vi "Laser Power Ctrl Ext Setup.vi"(0 "Wavelength":u16, 7 "Previous Path":path, 11 "Settings":string[](array[string])) -> (4 "Settings Out":string[](array[string]), 8 "Ext Ctrl Path":path, 15 "Canceled?":bool)   [LabVIEW 2020]
uses:
  <vilib>/Utility/miscctls.llb/LVPointTypeDef.ctl
panel:
  in  "Select Source":bool
  in  "Calling VI Ref":refnum<vi>
  in  "Cancel":bool
  in  "Done":bool
  in  "Setting 10":string
  in  "Setting 09":string
  in  "Setting 08":string
  in  "Setting 07":string
  in  "Setting 06":string
  in  "Setting 05":string
  in  "Setting 04":string
  in  "Setting 03":string
  in  "Setting 02":string
  in  "Setting 01":string
  out "External Power Control VI":string
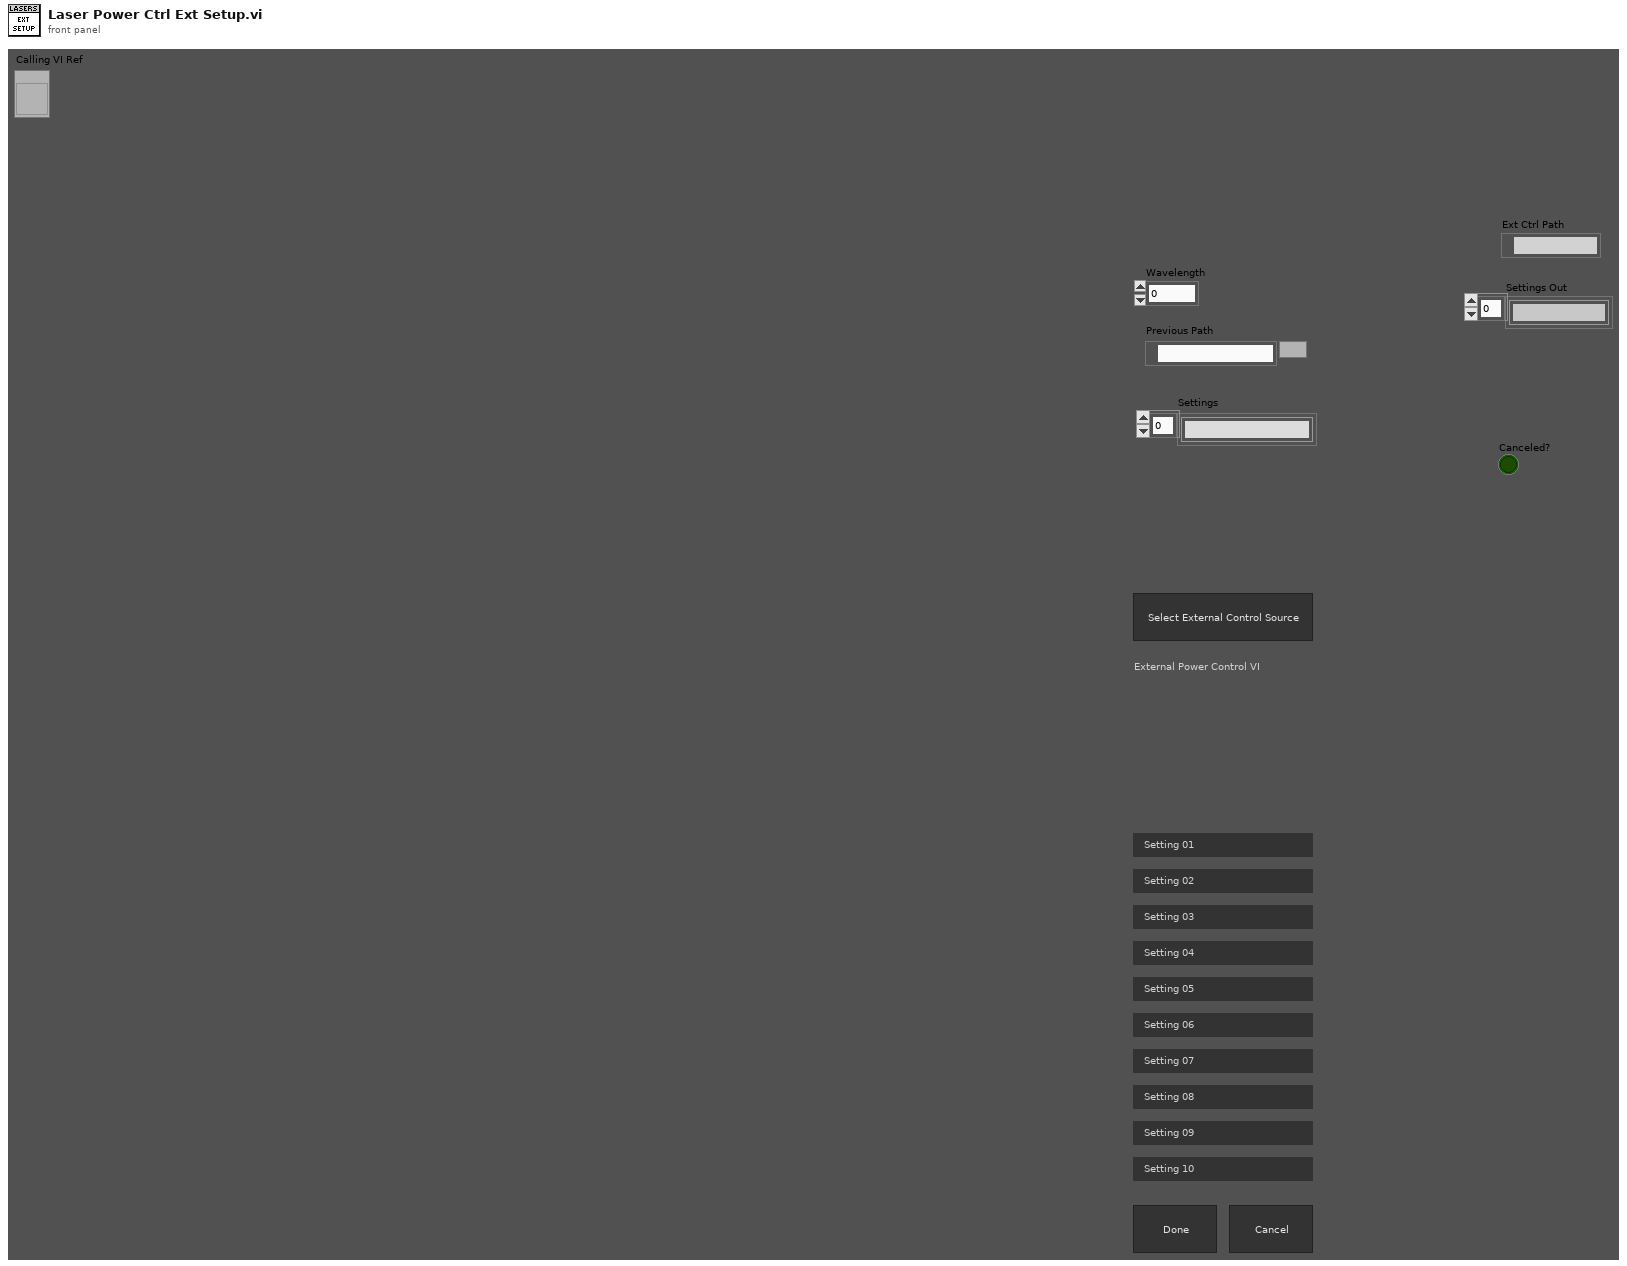
[diagram p1: front panel]
types:
  T1 = enum16{"Always On", "Always Off", "Off While Running"}
  T2 = typedef "LVPointTypeDef.ctl" = cluster{"Horizontal":i16, "Vertical":i16}
  T3 = typedef "LVRectTypeDef.ctl" = cluster{"Left":i16, "Top":i16, "Right":i16, "Bottom":i16}
  T4 = typedef "LVBoundsTypeDef.ctl" = cluster{"Width":u32, "Height":u32}
  T5 = enum8{"Enabled", "Disabled", "Disabled and Grayed Out"}
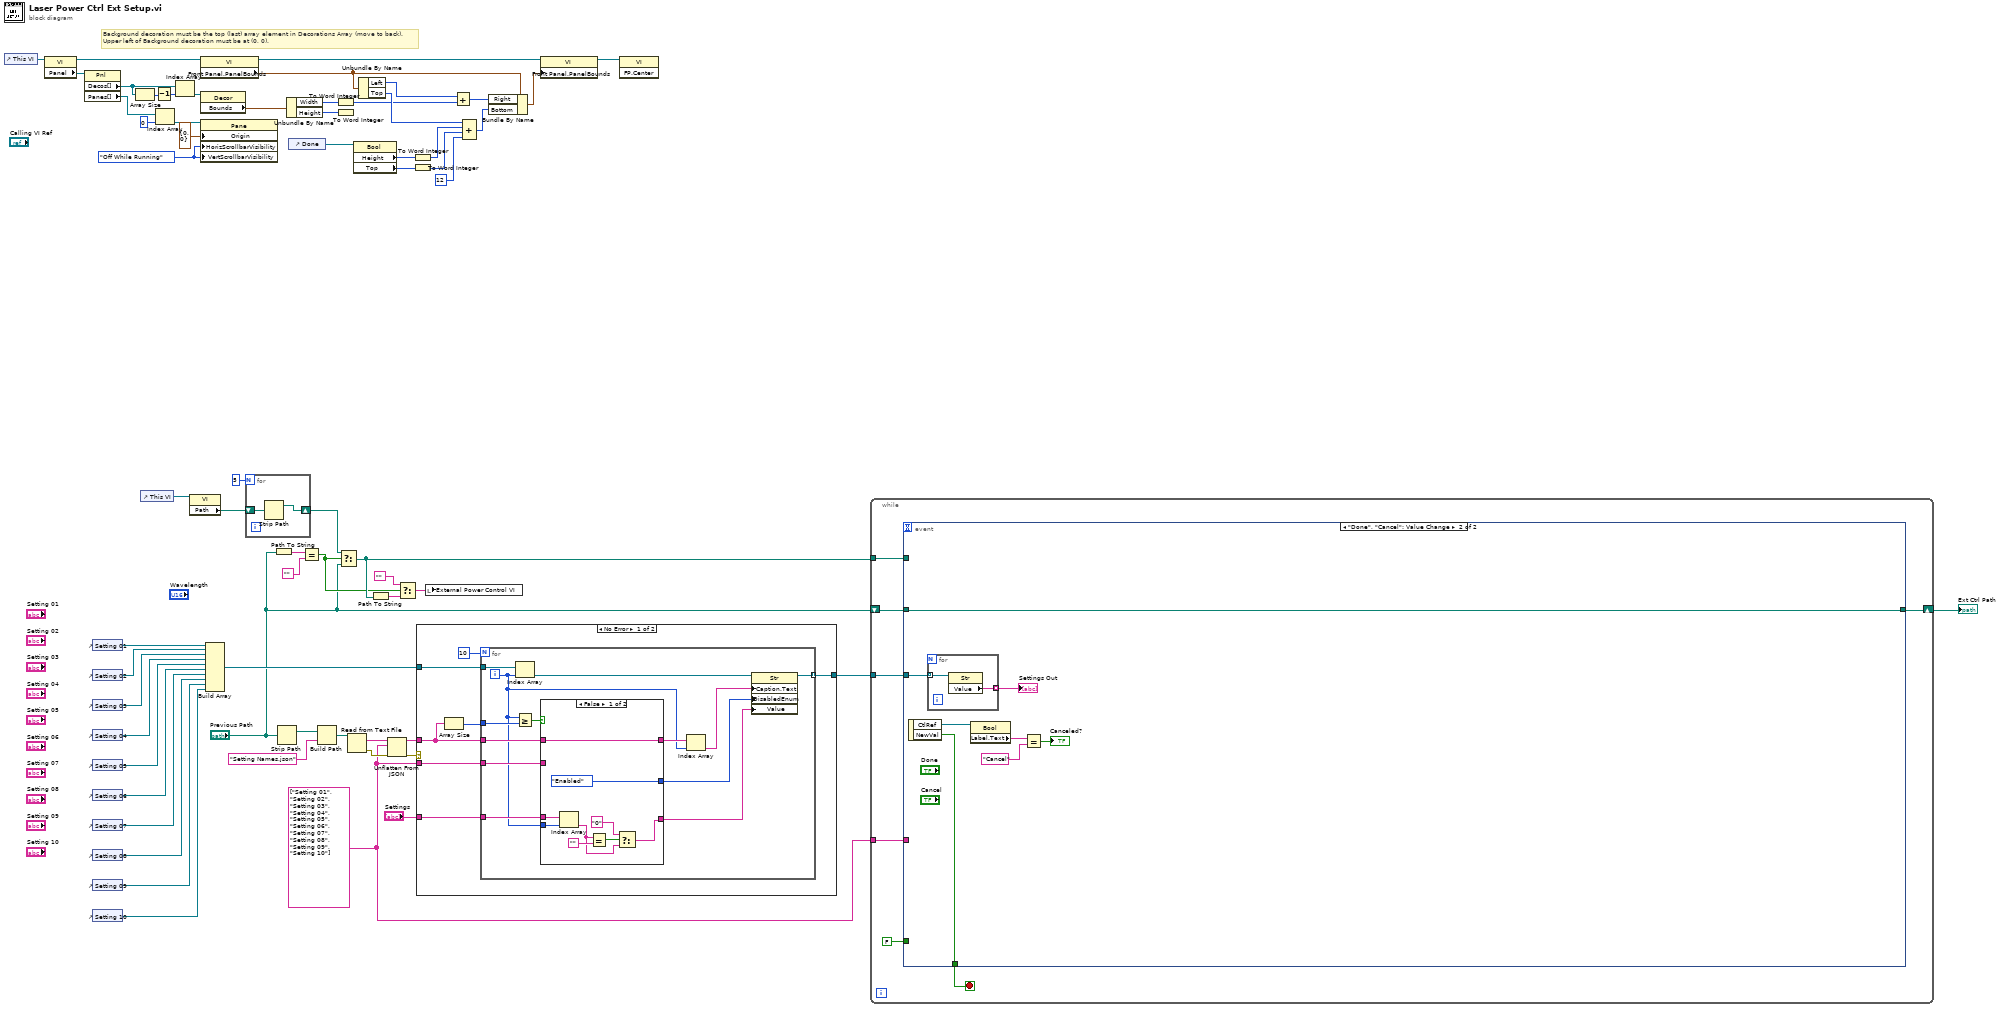
[diagram p0: block diagram]
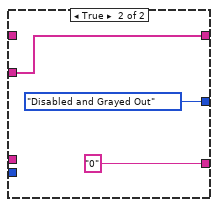
[diagram p2: hidden frame]
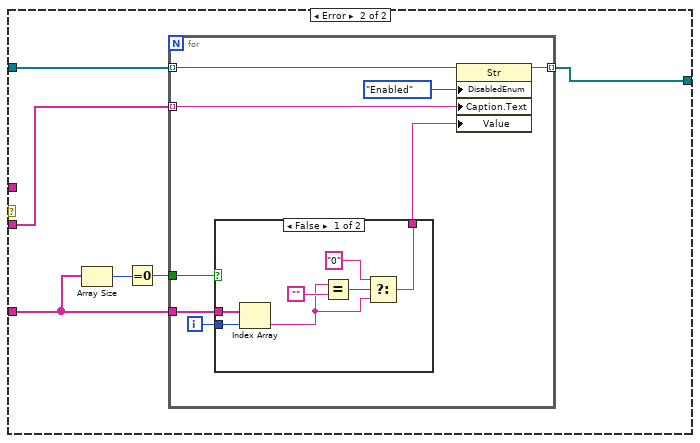
[diagram p3: hidden frame]
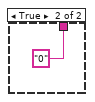
[diagram p4: hidden frame]
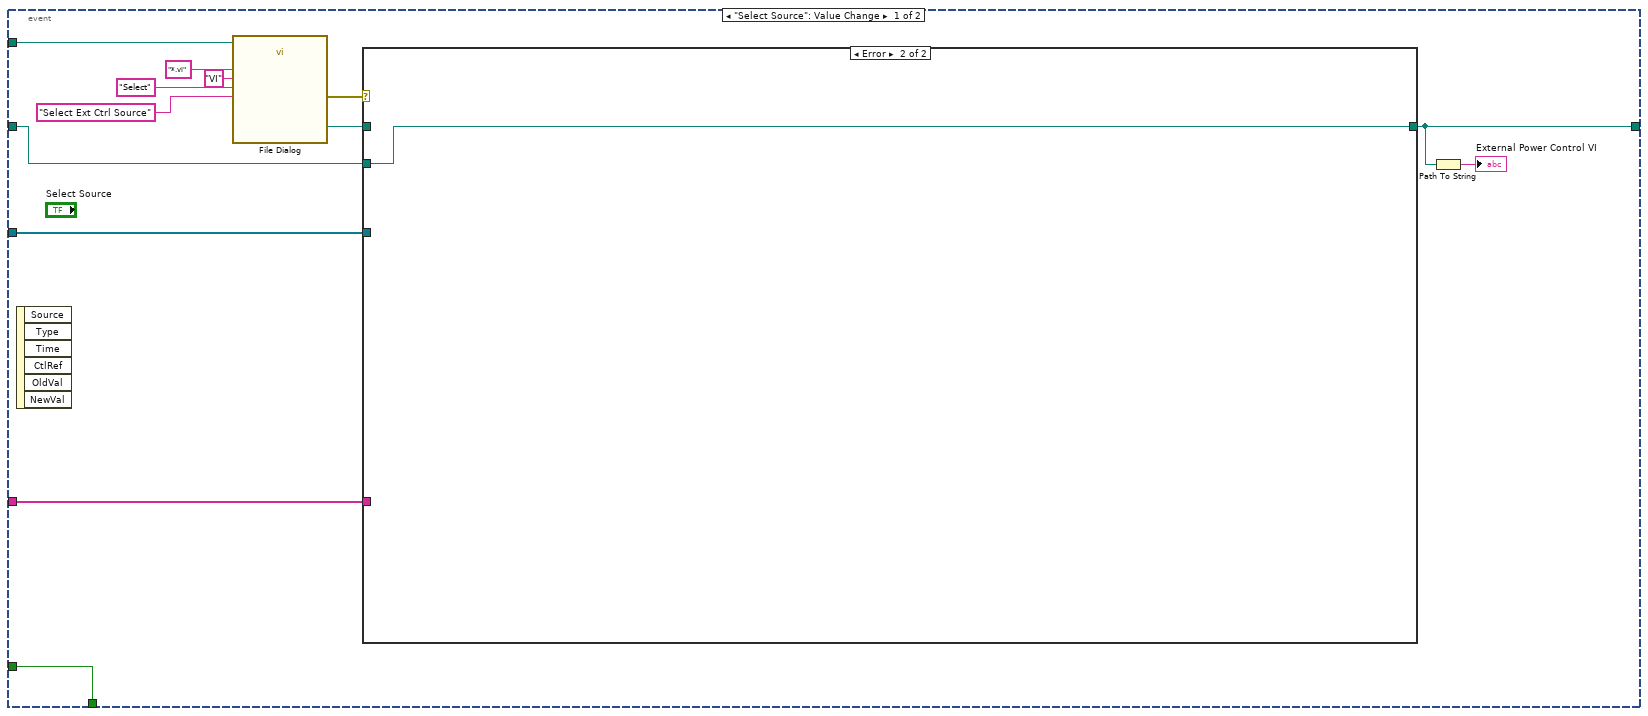
[diagram p5: hidden frame]
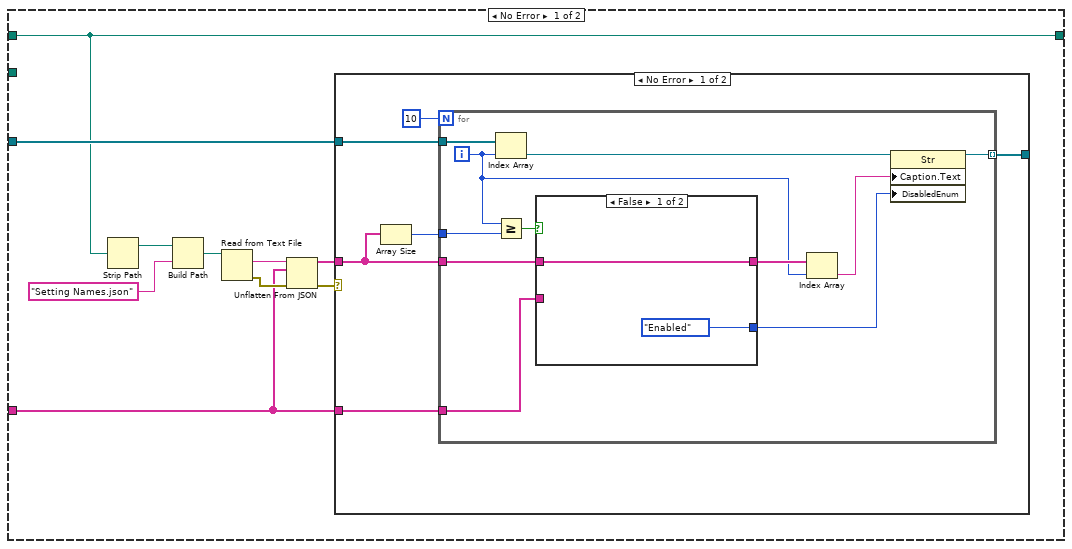
[diagram p6: hidden frame]
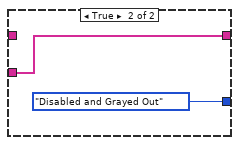
[diagram p7: hidden frame]
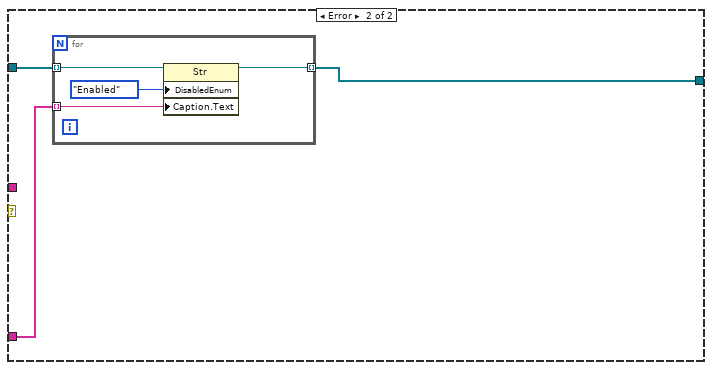
[diagram p8: hidden frame]
diagram:
  w11 = string[] ["Setting 01", "Setting 02", "Setting 03", "Setting 04", "Setting 05", "Setting 06", "Setting 07", "Setting 08", "Setting 09", "Setting 10"]
  w47 = T1."Off While Running" ("Vertical Scrollbar Visibility")
  # "Background decoration must be the top (last) array element in Decorations Array (move to back).\nUpper left of Background decoration must be at (0, 0)."
  n1 = control-ref of="This VI"() -> (w39:refnum<vi>)
  n2 = property class="VI"(reference=w39) -> (reference out=w48:refnum<vi>, "Panel"=w40:refnum<vi>)  [unwired: 1 in, 1 out]
  n3 = property class="Pnl"(reference=w40) -> ("Decos[]"=w38:refnum<vi>[], "Panes[]"=w44:refnum<vi>[])  [unwired: 1 in, 2 out]
  n4 = control-ref of="Setting 01"() -> (w30:refnum<vi>)
  n5 = control-ref of="Setting 02"() -> (w21:refnum<vi>)
  n6 = control-ref of="Setting 03"() -> (w22:refnum<vi>)
  n7 = control-ref of="Setting 04"() -> (w23:refnum<vi>)
  n8 = control-ref of="Setting 05"() -> (w24:refnum<vi>)
  n9 = control-ref of="Setting 06"() -> (w25:refnum<vi>)
  n10 = control-ref of="Setting 07"() -> (w26:refnum<vi>)
  n11 = control-ref of="Setting 08"() -> (w27:refnum<vi>)
  n12 = control-ref of="Setting 09"() -> (w28:refnum<vi>)
  n13 = control-ref of="Setting 10"() -> (w29:refnum<vi>)
  n14 = Array Size(array=w38) -> (size(s)=w36:i32)
  n15 = control-ref of="This VI"() -> (w16:refnum<vi>)
  n16 = Decrement(x=w36) -> (x-1=w37:i32)
  n17 = Index Array(array=w44, index=0) -> (element=w43:refnum<vi>)
  n18 = Index Array(array=w38, index=w37) -> (element=w46:refnum<vi>)
  n19 = property class="VI"(reference=w16) -> ("Path"=w15:path)  [unwired: 1 in, 2 out]
  n20 = property class="VI"(reference=w48) -> (reference out=w50:refnum<vi>, "Front Panel.PanelBounds"=w51:T3)  [unwired: 1 in, 1 out]
  n21 = property class="Decor"(reference=w46) -> ("Bounds"=w49:T4)  [unwired: 1 in, 2 out]
  n22 = property class="Pane"(reference=w43, "Origin"=T2 {"Horizontal"=0, "Vertical"=0}, "HorizScrollbarVisibility"=w47, "VertScrollbarVisibility"=w47) -> ()  [unwired: 1 in, 2 out]
  n23 = Build Array(w30, w21, w22, w23, w24, w25, w26, w27, w28, w29) -> (w20:refnum<vi>[])
  n24 = for {
    N: 5 -> [_]
    shift-right: [w65] -> w13
    shift-left: w15 -> [w66]
    n25 = Strip Path(path=w66) -> (stripped path=w65:path)  [unwired: 1 out]
  }
  n26 = Path To String(path="Previous Path") -> (string=w9:string)
  n27 = Strip Path(path="Previous Path") -> (stripped path=w35:path)  [unwired: 1 out]
  n28 = Unbundle By Name(w49) -> ("Width"=w54:u32, "Height"=w57:u32)
  n29 = control-ref of="Done"() -> (w41:refnum<vi>)
  n30 = Equal?(x=w9, y="") -> (x = y?=w8:bool)
  n31 = Build Path(base path=w35, name or relative path="Setting Names.json") -> (appended path=w33:path)
  n32 = To Word Integer(number=w54) -> (16bit integer=w56:i16)
  n33 = To Word Integer(number=w57) -> ()  [unwired: 1 out]
  n34 = Select(t=w13, s=w8, f="Previous Path") -> (s? t:f=w10:path)
  n35 = Read from Text File(file (use dialog)=w33) -> (text=w32:string, error out=w31:errorcluster)  [unwired: 3 in, 2 out]
  n36 = property class="Bool"(reference=w41) -> ("Height"=w59:u32, "Top"=w60:i32)  [unwired: 1 in, 2 out]
  n37 = Unbundle By Name(w51) -> ("Left"=w53:i16, "Top"=w64:i16)
  n38 = Path To String(path=w10) -> (string=w5:string)
  n39 = Unflatten From JSON(JSON string=w32, type and defaults=w11, error in (no error)=w31) -> (value=w19:string[], error out=w18:errorcluster)  [unwired: 4 in]
  n40 = Select(t="", s=w8, f=w5) -> (s? t:f=w4:string)
  n41 = To Word Integer(number=w59) -> (16bit integer=w62:i16)
  n42 = To Word Integer(number=w60) -> (16bit integer=w63:i16)
  n43 = case shown="No Error" w18 {
    tunnel: w20 -> [w73 w104]
    tunnel: w19 -> [w72 _]
    tunnel: w11 -> [w69 w103]
    tunnel: [w68 w102] -> w12
    tunnel: "Settings" -> [w67 w101]
    frame No Error {
      n44 = Array Size(array=w72) -> (size(s)=w71:i32)
      n45 = for {
        N: 10 -> [_]
        tunnel: w73 -> [w86]
        tunnel: w72 -> [w82]
        tunnel: w71 -> [w85]
        tunnel: w69 -> [w81]
        tunnel: [w77] -> w68 mode=indexing
        tunnel: w67 -> [w75]
        i -> [w74]
        n46 = Index Array(array=w86, index=w74) -> (element=w83:refnum<vi>)
        n47 = Greater Or Equal?(x=w74, y=w85) -> (x >= y?=w84:bool)
        n48 = case shown="False" w84 {
          tunnel: w82 -> [w95 _]
          tunnel: [w95 w98] -> w80
          tunnel: w81 -> [_ w98]
          tunnel: [T5."Enabled" ("Disabled") T5."Disabled and Grayed Out" ("Disabled")] -> w78
          tunnel: [w88 "0"] -> w76
          tunnel: w75 -> [w93 _]
          tunnel: w74 -> [w92 _]
          frame False {
            n49 = Index Array(array=w93, index=w92) -> (element=w89:string)
            n50 = Equal?(x=w89, y="") -> (x = y?=w90:bool)
            n51 = Select(t="0", s=w90, f=w89) -> (s? t:f=w88:string)
          }
          frame True {
          }
        }
        n52 = Index Array(array=w80, index=w74) -> (element=w79:string)
        n53 = property class="Str"(reference=w83, "Caption.Text"=w79, "DisabledEnum"=w78, "Value"=w76) -> (reference out=w77:refnum<vi>)  [unwired: 1 in, 1 out]
      }
    }
    frame Error {
      n54 = Array Size(array=w101) -> (size(s)=w100:i32)
      n55 = Equal To 0?(x=w100) -> (x = 0?=w99:bool)
      n56 = for {
        tunnel: w104 -> [w112] mode=indexing
        tunnel: w103 -> [w110] mode=indexing
        tunnel: [w109] -> w102 mode=indexing
        tunnel: w101 -> [w108]
        tunnel: w99 -> [w106]
        i -> [w105]
        n57 = case shown="False" w106 {
          tunnel: w108 -> [w115 _]
          tunnel: [w116 "0" ("String")] -> w107
          tunnel: w105 -> [w113 _]
          frame False {
            n58 = Index Array(array=w115, index=w113) -> (element=w114:string)
            n59 = Equal?(x=w114, y="") -> (x = y?=w118:bool)
            n60 = Select(t="0", s=w118, f=w114) -> (s? t:f=w116:string)
          }
          frame True {
          }
        }
        n61 = property class="Str"(reference=w112, "DisabledEnum"=T5."Enabled" ("Disabled"), "Caption.Text"=w110, "Value"=w107) -> (reference out=w109:refnum<vi>)  [unwired: 1 in, 1 out]
      }
    }
  }
  n62 = local write "External Power Control VI"(w4) -> ()
  n63 = Add(x=w53, y=w56) -> (x+y=w55:i16)
  n64 = Compound Arithmetic op=ADD(w64, w62, w63, i16 12 ("y")) -> (w58:i16)
  n65 = Bundle By Name(cluster=w51, "Right"=w55, "Bottom"=w58) -> (w52:T3)
  n66 = property class="VI"(reference=w50, "Front Panel.PanelBounds"=w52) -> (reference out=w17:refnum<vi>)  [unwired: 1 in, 1 out]
  n67 = invoke class="VI" method="FP.Center"(reference=w17) -> ()  [unwired: 2 in, 3 out]
  n68 = while {
    tunnel: w10 -> [w125]
    tunnel: w12 -> [w123]
    tunnel: w11 -> [w124]
    shift-right: [w121] -> w1
    shift-left: "Previous Path" -> [w122]
    stop <- w127 stop-if-true
    n69 = event shown="[1] \"Done\", \"Cancel\": Value Change" {
      selector: _ -> [_ _]
      dyn-events: _ -> [_ _]
      timeout: _ -> [_ _]
      tunnel: [w133 w184] -> w127
      tunnel: FALSE -> [w133 _]
      tunnel: w125 -> [w140 _]
      tunnel: w124 -> [w131 _]
      tunnel: w123 -> [w132 w182]
      tunnel: w122 -> [w130 w180]
      tunnel: [w129 w180] -> w121
      event "Select Source": Value Change {
        n70 = event-data() -> ()  [unwired: 1 in, 6 out]
        n71 = call "File Dialog"("start path"=w140, "prompt"="Select Ext Ctrl Source", "button label"="Select", "pattern (all files)"="*.vi", "pattern label"="VI") -> ("selected path"=w134:path, "error out"=w135:errorcluster)  [unwired: 7 in, 2 out]
        n72 = case shown="Error" w135 {
          tunnel: w134 -> [w141 _]
          tunnel: w132 -> [w143 _]
          tunnel: w131 -> [w142 _]
          tunnel: [w141 w179] -> w129
          tunnel: w130 -> [_ w179]
          frame No Error {
            n73 = Strip Path(path=w141) -> (stripped path=w150:path)  [unwired: 1 out]
            n74 = Build Path(base path=w150, name or relative path="Setting Names.json") -> (appended path=w148:path)
            n75 = Read from Text File(file (use dialog)=w148) -> (text=w147:string, error out=w146:errorcluster)  [unwired: 3 in, 2 out]
            n76 = Unflatten From JSON(JSON string=w147, type and defaults=w142, error in (no error)=w146) -> (value=w145:string[], error out=w144:errorcluster)  [unwired: 4 in]
            n77 = case shown="No Error" w144 {
              tunnel: w143 -> [w156 w174]
              tunnel: w145 -> [w155 _]
              tunnel: w142 -> [w152 w173]
              tunnel: [w151 w172] -> _
              frame No Error {
                n78 = Array Size(array=w155) -> (size(s)=w154:i32)
                n79 = for {
                  N: 10 -> [_]
                  tunnel: w156 -> [w167]
                  tunnel: w155 -> [w163]
                  tunnel: w154 -> [w166]
                  tunnel: w152 -> [w162]
                  tunnel: [w157] -> w151 mode=indexing
                  i -> [w160]
                  n80 = Index Array(array=w167, index=w160) -> (element=w164:refnum<vi>)
                  n81 = Greater Or Equal?(x=w160, y=w166) -> (x >= y?=w165:bool)
                  n82 = case shown="False" w165 {
                    tunnel: w163 -> [w169 _]
                    tunnel: [w169 w171] -> w161
                    tunnel: w162 -> [_ w171]
                    tunnel: [T5."Enabled" ("Disabled") T5."Disabled and Grayed Out" ("Disabled")] -> w158
                    frame False {
                    }
                    frame True {
                    }
                  }
                  n83 = Index Array(array=w161, index=w160) -> (element=w159:string)
                  n84 = property class="Str"(reference=w164, "Caption.Text"=w159, "DisabledEnum"=w158) -> (reference out=w157:refnum<vi>)  [unwired: 1 in, 1 out]
                }
              }
              frame Error {
                n85 = for {
                  tunnel: w174 -> [w178] mode=indexing
                  tunnel: w173 -> [w176] mode=indexing
                  tunnel: [w175] -> w172 mode=indexing
                  n86 = property class="Str"(reference=w178, "DisabledEnum"=T5."Enabled" ("Disabled"), "Caption.Text"=w176) -> (reference out=w175:refnum<vi>)  [unwired: 1 in, 1 out]
                }
              }
            }
          }
          frame Error {
          }
        }
        n87 = Path To String(path=w129) -> (string=→"External Power Control VI":string)
      }
      event "Done", "Cancel": Value Change {
        n88 = event-data() -> ("CtlRef"=w187:refnum<vi>, "NewVal"=w184:bool)  [unwired: 1 in]
        n89 = for {
          tunnel: w182 -> [w189] mode=indexing
          tunnel: [w188] -> w181 mode=indexing
          n90 = property class="Str"(reference=w189) -> ("Value"=w188:string)  [unwired: 1 in, 2 out]
        }
        "Settings Out" <- w181
        n91 = property class="Bool"(reference=w187) -> ("Label.Text"=w186:string)  [unwired: 1 in, 2 out]
        n92 = Equal?(x=w186, y="Cancel") -> (x = y?=→"Canceled?":bool)
      }
    }
  }
  "Ext Ctrl Path" <- w1
